vi "seconds since 1904 with units.vi"() -> (0 "seconds since 1Jan1904":dbl[unit] format="%.2f")   [LabVIEW 2012]
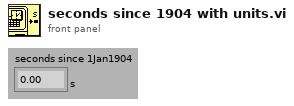
[diagram p1: front panel]
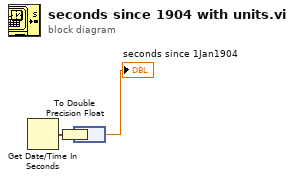
[diagram p0: block diagram]
diagram:
  n1 = Get Date/Time In Seconds() -> (seconds since 1Jan1904=w1:timestamp)
  n2 = To Double Precision Float(number=w1) -> (double precision float=w2:dbl)
  n3 = node(w2) -> (→"seconds since 1Jan1904":dbl[unit])
